vi "PCU_Set_SOP_Status.vi"(8 "error in (no error)":errorcluster, 10 "status":i32(ring) items=["LVP", "LHP", "LP45", "RCP", "LN45", "LCP"], 11 ".NET Reference in":refnum<k24>) -> (0 "error out":errorcluster, 3 "Reference out":refnum<k24>)   [LabVIEW 2017]
uses:
  D:/test/PDLSTS/LV_PDL LvVer17.0/LV_PDL_x86/DLL/InstrumentDLL.dll
  DLL/InstrumentDLL.dll
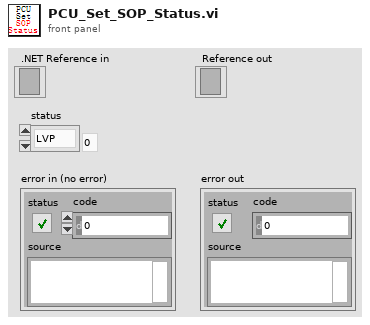
[diagram p1: front panel]
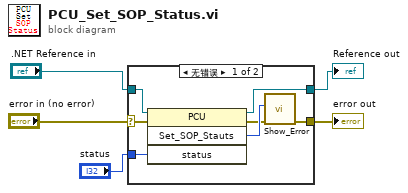
[diagram p0: block diagram]
diagram:
  n1 = case shown="无错误" "error in (no error)" {
    selector: "error in (no error)" -> [w9 w14]
    tunnel: ".NET Reference in" -> [w12 w13]
    tunnel: [w11 w13] -> w4
    tunnel: [w6 w14] -> w3
    tunnel: "status" -> [w10 _]
    frame No Error {
      n2 = invoke on="调用节点" class="PCU" method="Set_SOP_Stauts"(reference=w12, error in=w9, "status"=w10) -> (reference out=w11:refnum<k24>, error out=w7:errorcluster, "Set_SOP_Stauts"=w8:i32)  [unwired: 1 in, 1 out]
      n3 = call "Show_Error.vi"("error in (no error)"=w7, "Error"=w8) -> ("error out"=w6:errorcluster)  [unwired: 9 in]
    }
    frame Error {
    }
  }
  "Reference out" <- w4
  "error out" <- w3
